vi "Clusters.vi"() -> ()   [LabVIEW 2018]
uses:
  Control 1.ctl
panel:
  in  "Cluster 2":T1
  in  "Cluster":T1
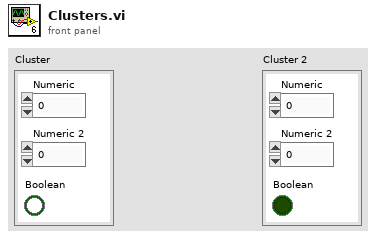
[diagram p1: front panel]
types:
  T1 = typedef "Control 1.ctl" = cluster{"Numeric":dbl, "Numeric 2":dbl, "Boolean":bool}
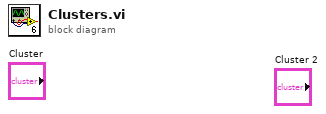
[diagram p0: block diagram]
diagram:
